vi "Begin.vi"(8 "error in":errorcluster) -> (0 "error out":errorcluster)   [LabVIEW 2018]
doc: "Called before other user functions, this VI is expected to open initial I/O refnums, load in file data, and do all program initialization. Notice that the <B>error out</B> terminal is simply used for data flow. Wiring it to other structures or subVIs ensures that this VI runs first."
uses:
  Right Motors.ctl
  Left Motors.ctl
  <vilib>/Rock Robotics/WPI/Joystick/WPI_JoystickDeviceEnum.ctl
  Joysticks.ctl
  <vilib>/Rock Robotics/WPI/ThirdParty/REV Robotics/SPARK MAX/Typedef/Spark MAX Motor Type.ctl
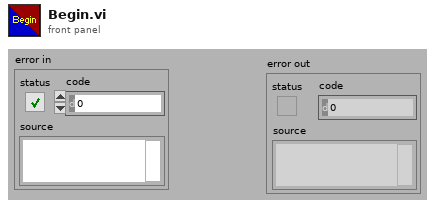
[diagram p1: front panel]
types:
  T1 = typedef "Joysticks.ctl" = enum16{"Joystick 1", "Joystick 2"}
  T2 = typedef "WPI_JoystickDeviceEnum.ctl" = enum16{"USB 0", "USB 1", "USB 2", "USB 3", "USB 4", "USB 5"}
  T3 = typedef "Left Motors.ctl" = enum16{"Left Motor 1", "Left Motor 2", "Left Motor 3"}
  T4 = typedef "Right Motors.ctl" = enum16{"Right Motor 1", "Right Motor 2", "Right Motor 3"}
  T5 = typedef "Spark MAX Motor Type.ctl" = enum16{"Brushed", "Brushless"}
  T6 = typedef "WPI_MotorControlDeviceRef.ctl" = cluster{"DeviceStatus":errorcluster, "Type":T7, "PWM":cluster{"PWM Channel":T8, "DeadBand":T9}, "CAN":cluster{"Device Number":u8, "SetOutput VI Ref":variant, "GetOutput VI Ref":variant, "Enable VI Ref":variant, "Disable VI Ref":variant, "Data":variant}, "Invert":bool, "DIO PWM":cluster{"PWM \"Enable\" Channel":T8, "DIOChannel":T10, "PWM Rate":dbl}}
  T7 = typedef "WPI_MotorControlType.ctl" = enum16{"PWM", "CAN", "DIO PWM"}
  T8 = typedef "FPGA_DIOPWMChannel.ctl" = enum8{"PWM 0", "PWM 1", "PWM 2", "PWM 3", "PWM 4", "PWM 5", "PWM 6", "PWM 7", "PWM 8", "PWM 9", "PWM MXP 0", "PWM MXP 1", "PWM MXP 2", "PWM MXP 3", "PWM MXP 4", "PWM MXP 5", "PWM MXP 6", "PWM MXP 7", "PWM MXP 8", "PWM MXP 9", "Invalid"}
  T9 = typedef "WPI_PWMDeadband.ctl" = cluster{"Name":string, "maxPositivePwm":i32, "minPositivePwm":i32, "centerPwm":i32, "maxNegativePwm":i32, "minNegativePwm":i32, "angularRange":u16}
  T10 = typedef "FPGA_DIOChannel.ctl" = enum8{"DIO 0", "DIO 1", "DIO 2", "DIO 3", "DIO 4", "DIO 5", "DIO 6", "DIO 7", "DIO 8", "DIO 9", "DIO MXP 0", "DIO MXP 1", "DIO MXP 2", "DIO MXP 3", "DIO MXP 4", "DIO MXP 5", "DIO MXP 6", "DIO MXP 7", "DIO MXP 8", "DIO MXP 9", "DIO MXP 10", "DIO MXP 11", "DIO MXP 12", "DIO MXP 13", "DIO MXP 14", "DIO MXP 15", "SPI Port CS1", "SPI Port CS2", "SPI Port CS3", "SPI Port MISO", "SPI Port MOSI", "Invalid"}
  T11 = typedef "WPI_JoystickDevRef.ctl" = cluster{"Device":T2}
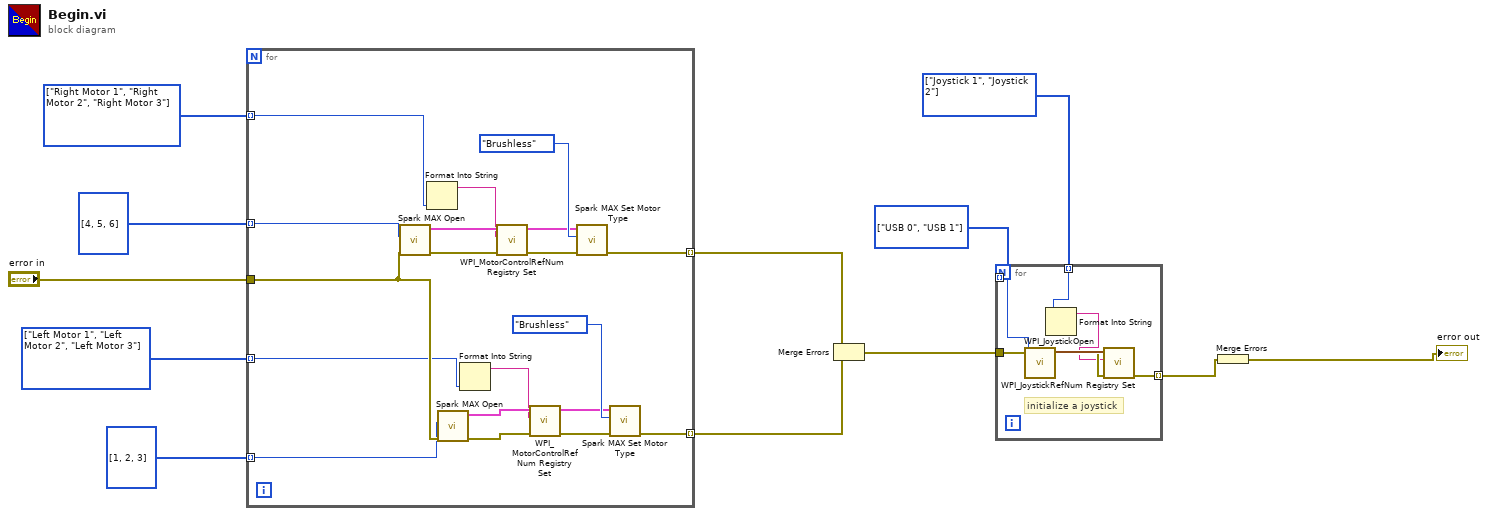
[diagram p0: block diagram]
diagram:
  w1 = T1[] [enum."Joystick 1", enum."Joystick 2"] items=["Joystick 1", "Joystick 2"]
  w5 = T2[] [enum."USB 0", enum."USB 1"] items=["USB 0", "USB 1", "USB 2", "USB 3", "USB 4", "USB 5"]
  w11 = T3[] [enum."Left Motor 1", enum."Left Motor 2", enum."Left Motor 3"] items=["Left Motor 1", "Left Motor 2", "Left Motor 3"]
  w10 = T4[] [enum."Right Motor 1", enum."Right Motor 2", enum."Right Motor 3"] items=["Right Motor 1", "Right Motor 2", "Right Motor 3"]
  n1 = for {
    tunnel: "error in" -> [w21]
    tunnel: w11 -> [w18] mode=indexing
    tunnel: w10 -> [w17] mode=indexing
    tunnel: u8[] [1, 2, 3] -> [w16] mode=indexing
    tunnel: u8[] [4, 5, 6] -> [w15] mode=indexing
    tunnel: [w14] -> w7 mode=indexing
    tunnel: [w13] -> w6 mode=indexing
    n2 = call <vilib>:"Spark MAX Open.vi"("error in (no error)"=w21, "Device Number"=w15) -> ("error out"=w28:errorcluster, "MotorControlDeviceRef"=w30:T6)  [unwired: 8 in]
    n3 = Format Into String(w17) -> (resulting string=w29:string)  [unwired: 3 in, 1 out]
    n4 = call <vilib>:"Spark MAX Open.vi"("error in (no error)"=w21, "Device Number"=w16) -> ("error out"=w20:errorcluster, "MotorControlDeviceRef"=w24:T6)  [unwired: 8 in]
    n5 = Format Into String(w18) -> (resulting string=w23:string)  [unwired: 3 in, 1 out]
    n6 = call <vilib>:"WPI_MotorControlRefNum Registry Set.vi"("error in (no error)"=w28, "refnum name"=w29, "MotorControlDevRef"=w30) -> ("error out"=w26:errorcluster, "MotorControlDevRef"=w27:T6)  [unwired: 7 in]
    n7 = call <vilib>:"WPI_MotorControlRefNum Registry Set.vi"("error in (no error)"=w20, "refnum name"=w23, "MotorControlDevRef"=w24) -> ("error out"=w19:errorcluster, "MotorControlDevRef"=w22:T6)  [unwired: 7 in]
    n8 = call <vilib>:"Spark MAX Set Motor Type.vi"("error in (no error)"=w26, "Enum"=Spark_MAX_Motor_Type."Brushless", "MotorControlDevRef"=w27) -> ("error out"=w13:errorcluster)  [unwired: 7 in, 1 out]
    n9 = call <vilib>:"Spark MAX Set Motor Type.vi"("error in (no error)"=w19, "Enum"=Spark_MAX_Motor_Type."Brushless", "MotorControlDevRef"=w22) -> ("error out"=w14:errorcluster)  [unwired: 7 in, 1 out]
  }
  n10 = Merge Errors(w6, w7) -> (w4:errorcluster)
  n11 = for {
    tunnel: w5 -> [w36] mode=indexing
    tunnel: w4 -> [w35]
    tunnel: [w34] -> w3 mode=indexing
    tunnel: w1 -> [w32] mode=indexing
    # "initialize a joystick"
    n12 = call <vilib>:"WPI_JoystickOpen.vi"("JoystickDevice"=w36) -> ("JoystickDevRef"=w37:T11)  [unwired: 10 in]
    n13 = Format Into String(w32) -> (resulting string=w33:string)  [unwired: 3 in, 1 out]
    n14 = call <vilib>:"WPI_JoystickRefNum Registry Set.vi"("error in (no error)"=w35, "refnum name"=w33, "JoystickDevRef"=w37) -> ("error out"=w34:errorcluster)  [unwired: 7 in, 1 out]
  }
  n15 = Merge Errors(w3) -> (→"error out":errorcluster)
